vi "LEIN m SIC Command N.vi"(11 "error in (no error)":errorcluster) -> (6 "queue out":refnum<queue>, 15 "error out":errorcluster)   [LabVIEW 2011]
uses:
  Defenitions/LEIN cycle holder.ctl
  Defenitions/LEIN CMD Cluster.ctl
  Defenitions/LEIN CMD List.ctl
  Defenitions/LEIN Reply Holder.ctl
  Defenitions/LEIN custom reply Q.ctl
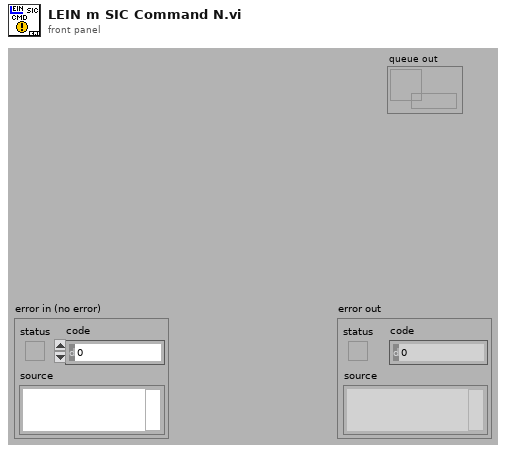
[diagram p1: front panel]
types:
  T1 = typedef "LEIN cycle holder.ctl" = cluster{"CMD":T2, "Retry if  unsucessful":bool, "LEIN reply holder":T4, "Reply in custom Q":bool, "LEIN custom reply Q":T5}
  T2 = typedef "LEIN CMD Cluster.ctl" = cluster{"SID":u8, "ANF":bool, "CMD":T3, "DATA":u8[]}
  T3 = typedef "LEIN CMD List.ctl" = enum8{"ACTI", "TASK", "RES0", "STAT", "RES1", "RES2", "RES3", "USER"}
  T4 = typedef "LEIN Reply Holder.ctl" = cluster{"Reply msg(cmdif no reply)":T2, "Reply time":timestamp, "Valid reply":bool}
  T5 = typedef "LEIN custom reply Q.ctl" = refnum<queue>
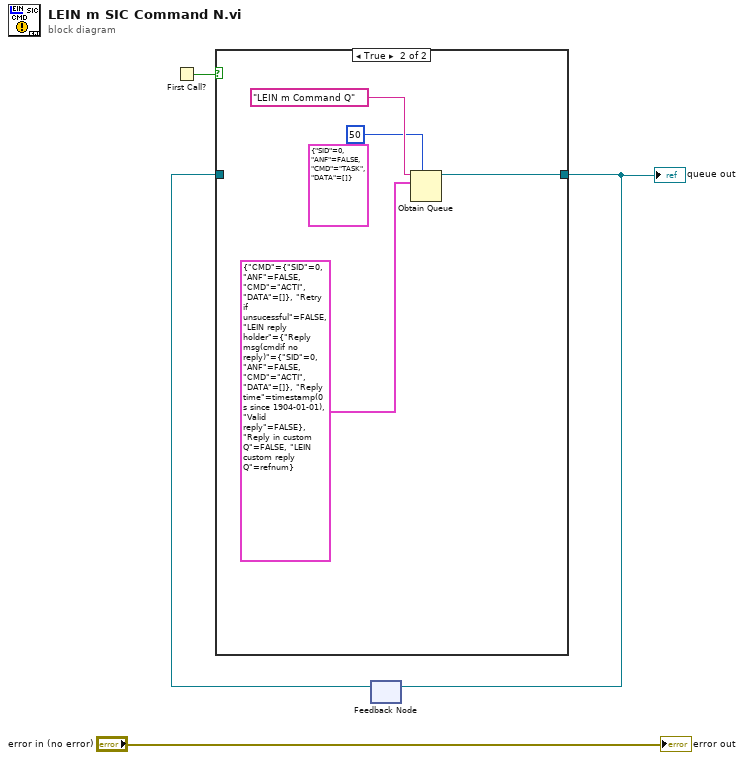
[diagram p0: block diagram]
diagram:
  n1 = First Call?() -> (First Call?: T/F=w3:bool)
  n2 = feedback #1() -> (w1:refnum<queue>)  [unwired: 1 in]
  n3 = case shown="True" w3 {
    tunnel: [w5 w7] -> w2
    tunnel: w1 -> [w5 _]
    frame False {
    }
    frame True {
      (unwired) T2 {"SID"=0, "ANF"=FALSE, "CMD"=enum."TASK", "DATA"=[]} ("CMD")
      n4 = Obtain Queue(max queue size (-1, unlimited)=50, name (unnamed)="LEIN m Command Q", element data type=T1 {"CMD"={"SID"=0, "ANF"=FALSE, "CMD"=enum."ACTI", "DATA"=[]}, "Retry if  unsucessful"=FALSE, "LEIN reply holder"={"Reply msg(cmdif no reply)"={"SID"=0, "ANF"=FALSE, "CMD"=enum."ACTI", "DATA"=[]}, "Reply time"=timestamp(0 s since 1904-01-01), "Valid reply"=FALSE}, "Reply in custom Q"=FALSE, "LEIN custom reply Q"=refnum} ("element")) -> (queue out=w7:refnum<queue>)  [unwired: 2 in, 2 out]
    }
  }
  "queue out" <- w2
  n5 = feedback-in #1(w2) -> ()
  "error out" <- "error in (no error)"
